vi "test_Basic Waveform Read and Write.vi"(8 "error in (no error)":errorcluster, 11 "DMA Channels Basic Testing in":refnum<class "DMA Channels Basic Testing.lvclass">) -> (0 "error out":errorcluster, 3 "DMA Channels Basic Testing out":refnum<class "DMA Channels Basic Testing.lvclass">)   [LabVIEW 2018, in "DMA Channels Basic Testing.lvclass"]
uses:
  DMA Channels Basic Testing.lvclass
panel:
  out "Waveform 2":waveform(dbl)(graph)
  out "Waveform 1":waveform(dbl)(graph)
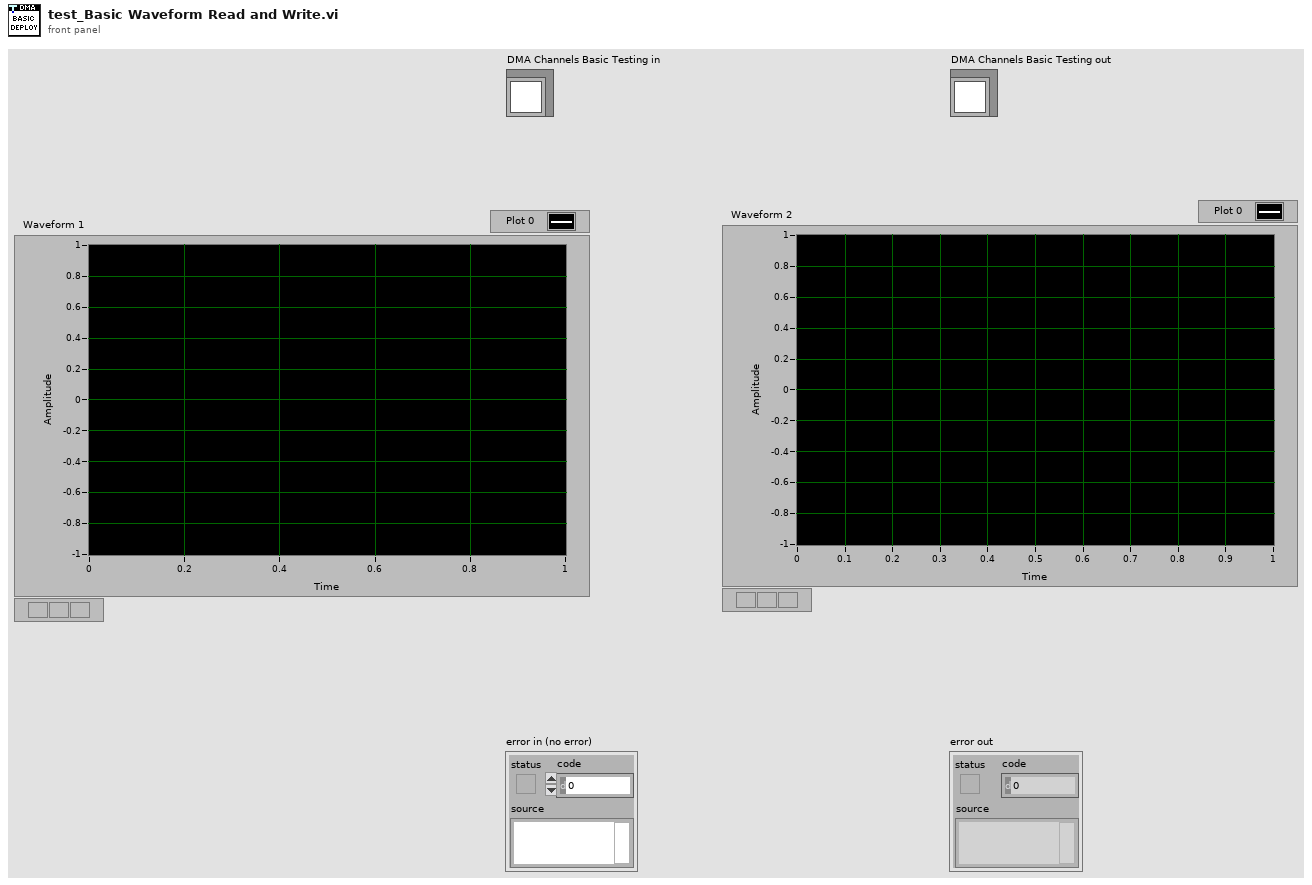
[diagram p1: front panel]
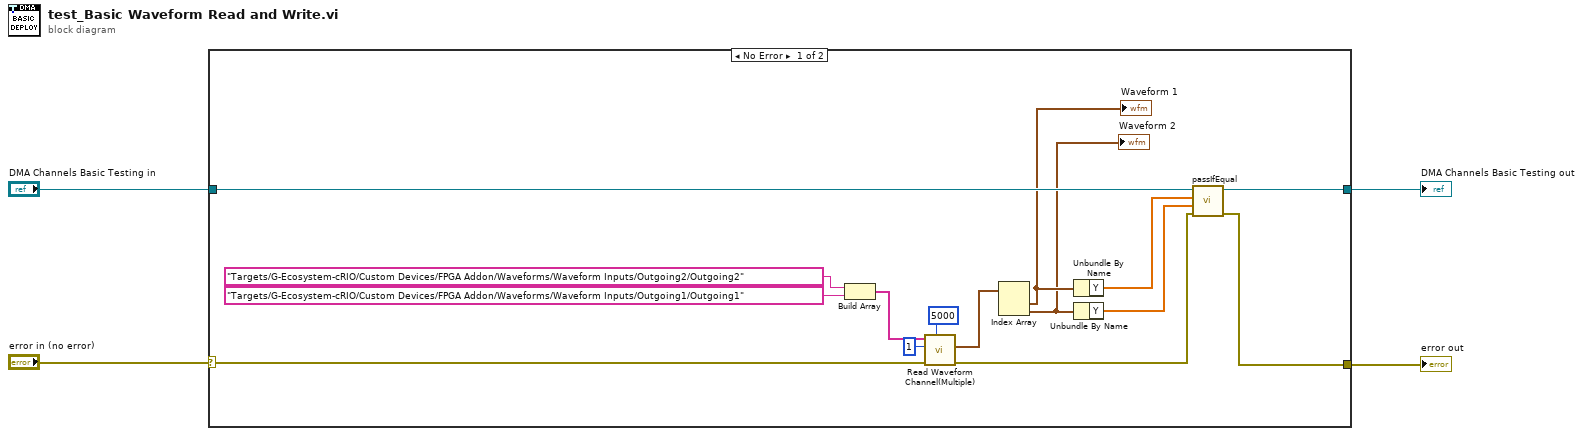
[diagram p0: block diagram]
diagram:
  n1 = case shown="No Error" "error in (no error)" {
    selector: "error in (no error)" -> [w14 w20]
    tunnel: "DMA Channels Basic Testing in" -> [w17 w21]
    tunnel: [w15 w21] -> w1
    tunnel: [w16 w20] -> w3
    frame No Error {
      n2 = Build Array("Targets/G-Ecosystem-cRIO/Custom Devices/FPGA Addon/Waveforms/Waveform Inputs/Outgoing2/Outgoing2" ("waveform path"), "Targets/G-Ecosystem-cRIO/Custom Devices/FPGA Addon/Waveforms/Waveform Inputs/Outgoing1/Outgoing1" ("waveform path")) -> (w10:string[])
      n3 = call "Read Waveform Channel(Multiple).vi"("Timeout"=5000, "error in (no error)"=w14, "Number of Reads"=1, "Waveform Paths in"=w10) -> ("error out"=w8:errorcluster, "Waveform Data"=w9:waveform(dbl)[])  [unwired: 5 in, 1 out]
      n4 = Index Array(array=w9) -> (element #1=w7:waveform(dbl), element #2=w6:waveform(dbl))  [unwired: 2 in]
      "Waveform 1" <- w7
      "Waveform 2" <- w6
      n5 = Unbundle By Name(w7) -> ("Y"=w19:dbl[])
      n6 = Unbundle By Name(w6) -> ("Y"=w18:dbl[])
      n7 = call-dynamic "passIfEqual.vi"("error in (no error)"=w8, "y"=w18, "x"=w19, "TestCase in"=w17) -> ("error out"=w16:errorcluster, "TestCase out"=w15:refnum<class "DMA Channels Basic Testing.lvclass">)  [unwired: 6 in]
    }
    frame Error {
    }
  }
  "error out" <- w3
  "DMA Channels Basic Testing out" <- w1
